vi "序号清零子vi.vi"() -> (3 "当日序号":string)   [LabVIEW 2014]
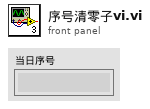
[diagram p1: front panel]
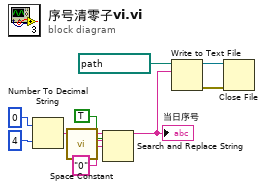
[diagram p0: block diagram]
diagram:
  n1 = Number To Decimal String(number=0 ("数字"), width (-)=i16 4 ("宽度(-)")) -> (decimal integer string=w9:string)
  n2 = call <vilib>:"Space Constant.vi"() -> ("String"=w6:string)
  n3 = Search and Replace String(replace all?=TRUE ("替换全部？(F)"), input string=w9, search string=w6, replace string="0" ("替换字符串(\"\")")) -> (result string=w1:string)  [unwired: 4 in, 3 out]
  "当日序号" <- w1
  n4 = Write to Text File(file (use dialog)=path "D:/序号.txt" ("文件（使用对话框）"), text=w1) -> (refnum out=w3:refnum<file>, error out=w2:errorcluster)  [unwired: 2 in, 1 out]
  n5 = Close File(refnum=w3, error in=w2) -> ()  [unwired: 2 out]
